vi "Encoded String To UTF-8.vi"(8 "error in (no error)":errorcluster, 10 "Encoded string":string, 11 "Encoding in":refnum<class "CConfig Automatic Encoding.lvclass">) -> (0 "error out":errorcluster, 2 "UTF-8 string":string, 3 "Encoding out":refnum<class "CConfig Automatic Encoding.lvclass">)   [LabVIEW 2013, in "CConfig Automatic Encoding.lvclass"]
doc: "Copyright 2018, Carya Automatisering, Wiebe Walstra."
uses:
  CConfig Automatic Encoding.lvclass
  CConfig Automatic Encoding.lvclass/CConfig Automatic Encoding.ctl
  CConfig Encoding.lvclass
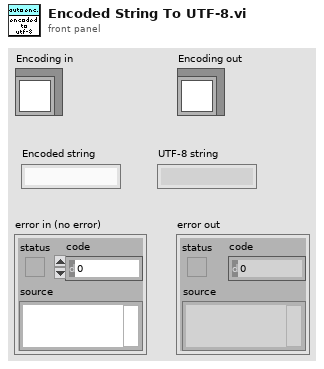
[diagram p1: front panel]
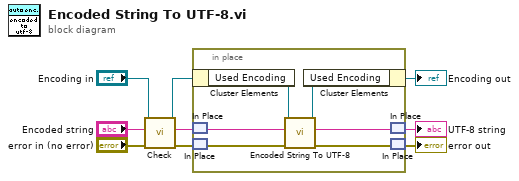
[diagram p0: block diagram]
diagram:
  n1 = call-dynamic "Check.vi"("error in (no error)"="error in (no error)", "Encoded string"="Encoded string", "Encoding in"="Encoding in") -> ("error out"=w4:errorcluster, "Encoded string"=w2:string, "Encoding out"=w6:refnum<class "CConfig Automatic Encoding.lvclass">)  [unwired: 5 in, 1 out]
  n2 = in-place {
    n3 = in-place-cluster #1(w6) -> ("Used Encoding"=w15:refnum<class "CConfig Encoding.lvclass">)
    n4 = in-place-match #2(w2) -> (w11:string)
    n5 = in-place-match #3(w4) -> (w13:errorcluster)
    n6 = call-dynamic "Encoded String To UTF-8.vi"("error in (no error)"=w13, "Encoded string"=w11, "Encoding in"=w15) -> ("error out"=w12:errorcluster, "UTF-8 string"=w10:string, "Encoding out"=w14:refnum<class "CConfig Encoding.lvclass">)  [unwired: 6 in]
    n7 = in-place-cluster #1("Used Encoding"=w14) -> (→"Encoding out":refnum<class "CConfig Automatic Encoding.lvclass">)
    n8 = in-place-match #2(w10) -> (→"UTF-8 string":string)
    n9 = in-place-match #3(w12) -> (→"error out":errorcluster)
  }
